vi "Relay Control.vi"(0 "GEA2 Reference In":refnum<k24>, 5 "Relay":enum16{"Motor Enable", "Valve", "Both"}(ring), 7 "State":enum16{"On", "Off"}(ring), 11 "Error In":errorcluster) -> (4 "GEA2 Reference Out":refnum<k24>, 6 "Pass/Fail?":bool, 8 "Report Text":string, 15 "Error Out":errorcluster)   [LabVIEW 2018, in "TLMB.lvlib"]
doc: "Use this VI to control the state of the motor enable and valve relay."
uses:
  Projects/TLMB.lvlib
  D:/Common/LabVIEW GEA2 Toolkit/source/GEA3 DLL Source/GeaCommunication.dll
  Common/LabVIEW GEA2 Toolkit/source/GEA3 DLL Source/GeaCommunication.dll
  Common/LabVIEW GEA2 Toolkit/GEA3/type defs/Source_Destination.ctl
  Common/LabVIEW GEA2 Toolkit/GEA3/type defs/ERD Read Data In.ctl
  Common/LabVIEW GEA2 Toolkit/GEA3/type defs/Data Type.ctl
  Common/LabVIEW GEA2 Toolkit/GEA3/type defs/ERD Write Data In.ctl
  C:/Users/iallatyp/Desktop/New folder/GEA3/library/GEA2_Toolkit.lvlib
panel:
  in  "Standalone?":bool
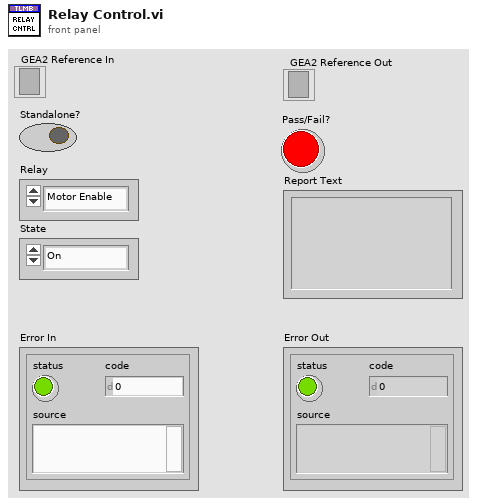
[diagram p1: front panel]
types:
  T1 = typedef "GEA2_Toolkit.lvlib/Source_Destination.ctl" = cluster{"Source":u8, "Destination":u8}
  T2 = typedef "GEA2_Toolkit.lvlib/ERD Write Data In.ctl" = cluster{"ERD Number":u16, "Data Type":T3, "Data":string}
  T3 = typedef "GEA2_Toolkit.lvlib/Data Type.ctl" = enum16{"string", "boolean", "uint8_t", "uint16_t", "uint32_t", "uint64_t", "int8_t", "int16_t", "int32_t", "int64_t"}
  T4 = typedef "GEA2_Toolkit.lvlib/ERD Read Data In.ctl" = cluster{"ERD Number":u16, "Data Type":T3}
  T5 = typedef "GEA2_Toolkit.lvlib/ERD Read Data Out.ctl" = cluster{"ERD Number":u16, "Data":string}
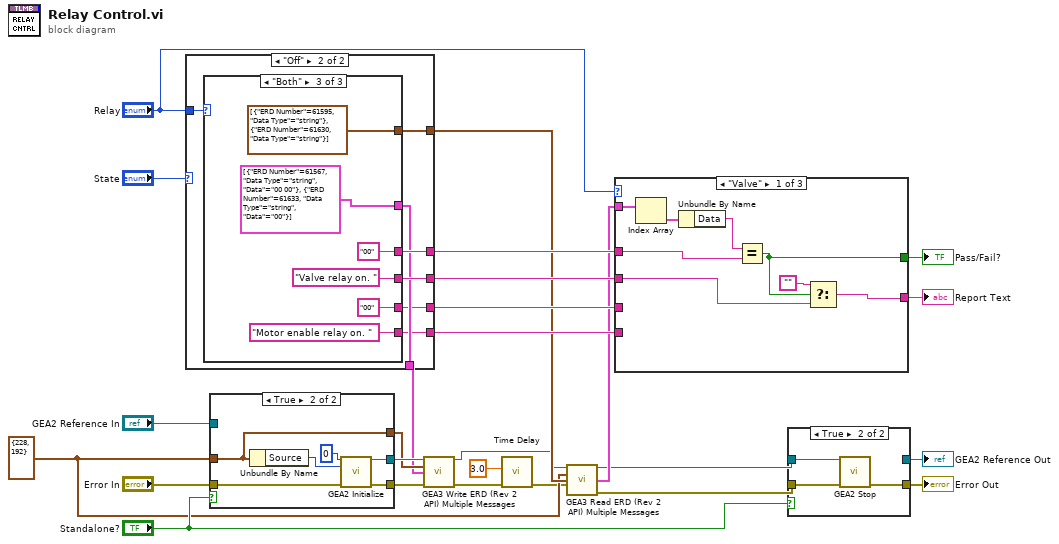
[diagram p0: block diagram]
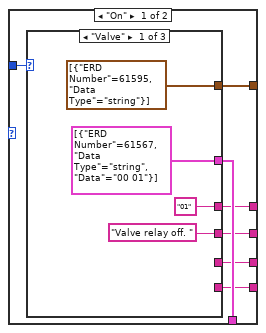
[diagram p2: hidden frame]
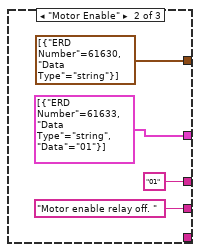
[diagram p3: hidden frame]
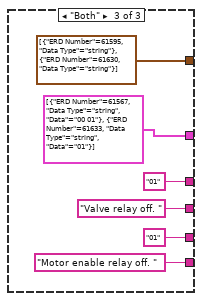
[diagram p4: hidden frame]
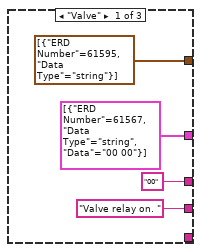
[diagram p5: hidden frame]
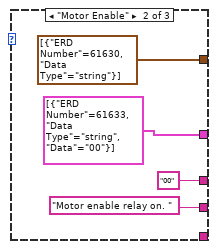
[diagram p6: hidden frame]
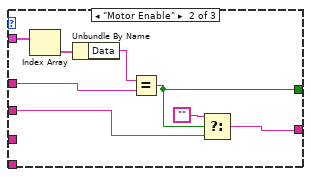
[diagram p7: hidden frame]
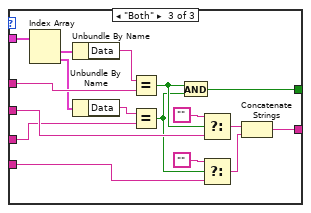
[diagram p8: hidden frame]
diagram:
  w11 = T1 {"Source"=228, "Destination"=192} ("GEA Inputs")
  n1 = case shown="\"Off\"" "State" {
    tunnel: [w33 w51] -> w4
    tunnel: [w32 w53] -> w19
    tunnel: [w31 w52] -> w18
    tunnel: [w30 w54] -> w12
    tunnel: "Relay" -> [w29 w50]
    tunnel: [w27 w49] -> w15
    tunnel: [w28 w48] -> w14
    frame "On" {
      n2 = case shown="\"Valve\"" w29 {
        tunnel: [T2[] [{"ERD Number"=61567, "Data Type"=enum."string", "Data"="00 01"}] ("Write ERD List") T2[] [{"ERD Number"=61633, "Data Type"=enum."string", "Data"="01"}] ("Write ERD List") T2[] [{"ERD Number"=61567, "Data Type"=enum."string", "Data"="00 01"}, {"ERD Number"=61633, "Data Type"=enum."string", "Data"="01"}] ("Write ERD List")] -> w33
        tunnel: ["01" ("y") "01" ("y") "01" ("y")] -> w32
        tunnel: ["Valve relay off. " ("f") "Motor enable relay off. " ("f") "Valve relay off. " ("f")] -> w31
        tunnel: [T4[] [{"ERD Number"=61595, "Data Type"=enum."string"}] ("Read ERD List") T4[] [{"ERD Number"=61630, "Data Type"=enum."string"}] ("Read ERD List") T4[] [{"ERD Number"=61595, "Data Type"=enum."string"}, {"ERD Number"=61630, "Data Type"=enum."string"}] ("Read ERD List")] -> w30
        tunnel: [_ _ "01" ("y")] -> w28
        tunnel: [_ _ "Motor enable relay off. " ("f")] -> w27
        frame "Valve" {
        }
        frame "Motor Enable" {
        }
        frame "Both" {
        }
      }
    }
    frame "Off" {
      n3 = case shown="\"Both\"" w50 {
        tunnel: [T2[] [{"ERD Number"=61567, "Data Type"=enum."string", "Data"="00 00"}] ("Write ERD List") T2[] [{"ERD Number"=61633, "Data Type"=enum."string", "Data"="00"}] ("Write ERD List") T2[] [{"ERD Number"=61567, "Data Type"=enum."string", "Data"="00 00"}, {"ERD Number"=61633, "Data Type"=enum."string", "Data"="00"}] ("Write ERD List")] -> w51
        tunnel: ["00" ("y") "00" ("y") "00" ("y")] -> w53
        tunnel: ["Valve relay on. " ("f") "Motor enable relay on. " ("f") "Valve relay on. " ("f")] -> w52
        tunnel: [T4[] [{"ERD Number"=61595, "Data Type"=enum."string"}] ("Read ERD List") T4[] [{"ERD Number"=61630, "Data Type"=enum."string"}] ("Read ERD List") T4[] [{"ERD Number"=61595, "Data Type"=enum."string"}, {"ERD Number"=61630, "Data Type"=enum."string"}] ("Read ERD List")] -> w54
        tunnel: [_ _ "Motor enable relay on. " ("f")] -> w49
        tunnel: [_ _ "00" ("y")] -> w48
        frame "Valve" {
        }
        frame "Motor Enable" {
        }
        frame "Both" {
        }
      }
    }
  }
  n4 = case shown="True" "Standalone?" {
    tunnel: "Error In" -> [w70 w75]
    tunnel: [w70 w73] -> w3
    tunnel: "GEA2 Reference In" -> [w71 _]
    tunnel: [w71 w74] -> w6
    tunnel: w11 -> [w69 w72]
    tunnel: [w69 w72] -> w5
    frame False {
    }
    frame True {
      n5 = Unbundle By Name(w72) -> ("Source"=w76:u8)
      n6 = call "GEA2 Initialize.vi"("Board Index"=0, "Source Address"=w76, "error in"=w75) -> ("GEA2 Reference Out"=w74:refnum<k24>, "error out"=w73:errorcluster)  [unwired: 10 in, 1 out]
    }
  }
  n7 = call "GEA3 Write ERD (Rev 2 API) Multiple Messages.vi"("GEA2 Reference In"=w6, "GEA Inputs"=w5, "Write ERD List"=w4, "Error In"=w3) -> ("GEA2 Reference Out"=w1:refnum<k24>, "Error Out"=w2:errorcluster)  [unwired: 9 in, 1 out]
  n8 = call "Time Delay"("error in (no error)"=w2, "Delay Time (s)"=3.0) -> ("error out"=w10:errorcluster)  [unwired: 9 in]
  n9 = call "GEA3 Read ERD (Rev 2 API) Multiple Messages.vi"("GEA2 Reference In"=w1, "GEA Inputs"=w11, "Read ERD List"=w12, "Error In"=w10) -> ("GEA2 Reference Out"=w8:refnum<k24>, "ERD Data Out"=w9:T5[], "Error Out"=w7:errorcluster)  [unwired: 8 in, 1 out]
  n10 = case shown="\"Valve\"" "Relay" {
    tunnel: [w84 w92 w96] -> w21
    tunnel: w9 -> [w83 w91 w109]
    tunnel: [w80 w88 w97] -> w20
    tunnel: w19 -> [w79 w86 w106]
    tunnel: w18 -> [w78 w87 w105]
    tunnel: w15 -> [_ _ w101]
    tunnel: w14 -> [_ _ w100]
    frame "Valve" {
      n11 = Index Array(array=w83) -> (element=w82:T5)  [unwired: 1 in]
      n12 = Unbundle By Name(w82) -> ("Data"=w81:string)
      n13 = Equal?(x=w81, y=w79) -> (x = y?=w80:bool)
      n14 = Select(t="", s=w80, f=w78) -> (s? t:f=w84:string)
    }
    frame "Motor Enable" {
      n15 = Index Array(array=w91) -> (element=w90:T5)  [unwired: 1 in]
      n16 = Unbundle By Name(w90) -> ("Data"=w89:string)
      n17 = Equal?(x=w89, y=w86) -> (x = y?=w88:bool)
      n18 = Select(t="", s=w88, f=w87) -> (s? t:f=w92:string)
    }
    frame "Both" {
      n19 = Index Array(array=w109) -> (element #1=w108:T5, element #2=w103:T5)  [unwired: 2 in]
      n20 = Unbundle By Name(w108) -> ("Data"=w107:string)
      n21 = Unbundle By Name(w103) -> ("Data"=w104:string)
      n22 = Equal?(x=w107, y=w106) -> (x = y?=w99:bool)
      n23 = Equal?(x=w104, y=w100) -> (x = y?=w98:bool)
      n24 = And(x=w99, y=w98) -> (x .and. y?=w97:bool)
      n25 = Select(t="", s=w99, f=w105) -> (s? t:f=w95:string)
      n26 = Select(t="", s=w98, f=w101) -> (s? t:f=w94:string)
      n27 = Concatenate Strings(w95, w94) -> (w96:string)
    }
  }
  "Pass/Fail?" <- w20
  "Report Text" <- w21
  n28 = case shown="True" "Standalone?" {
    tunnel: w7 -> [w112 w113]
    tunnel: [w112 w114] -> w26
    tunnel: [w111 _] -> w25
    tunnel: w8 -> [w111 w115]
    frame False {
    }
    frame True {
      n29 = call "GEA2 Stop.vi"("GEA2 Reference In"=w115, "Error In"=w113) -> ("Error Out"=w114:errorcluster)  [unwired: 13 in]
    }
  }
  "Error Out" <- w26
  "GEA2 Reference Out" <- w25
